vi "full adder.vi"() -> ()   [LabVIEW 2012]
panel:
  out "carry":bool
  out "sum":bool
  in  "c":bool
  in  "b":bool
  in  "a":bool
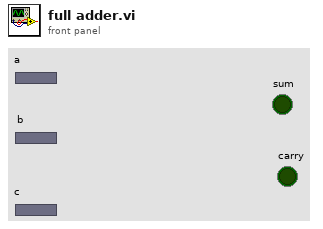
[diagram p1: front panel]
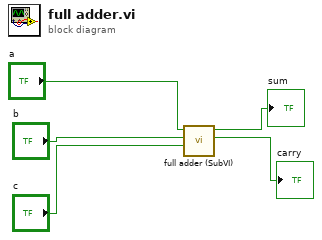
[diagram p0: block diagram]
diagram:
  n1 = call "full adder (SubVI).vi"("c"="c", "b"="b", "a"="a") -> ("carry"=→"carry":bool, "sum"=→"sum":bool)  [unwired: 7 in]
